vi "ClientIndividualUDP.vi"(0 "UDP Connection ID":refnum<k16>, 1 "Rover Inputs":cluster{"Left PWM":i32, "Right PWM":i32}={"Left PWM"=1500, "Right PWM"=1500}, 2 "Remote Port #":i32=61540, 3 "error in (no error)":errorcluster, 4 "Robot Symbol":string) -> (5 "connection ID out":refnum<k16>, 6 "Robot Heading":i32, 7 "error out":errorcluster)   [LabVIEW 2012]
panel:
  out "concatenated string":string
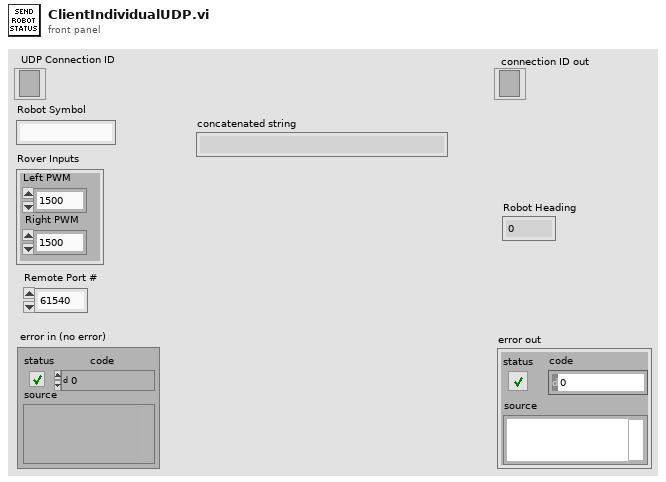
[diagram p1: front panel]
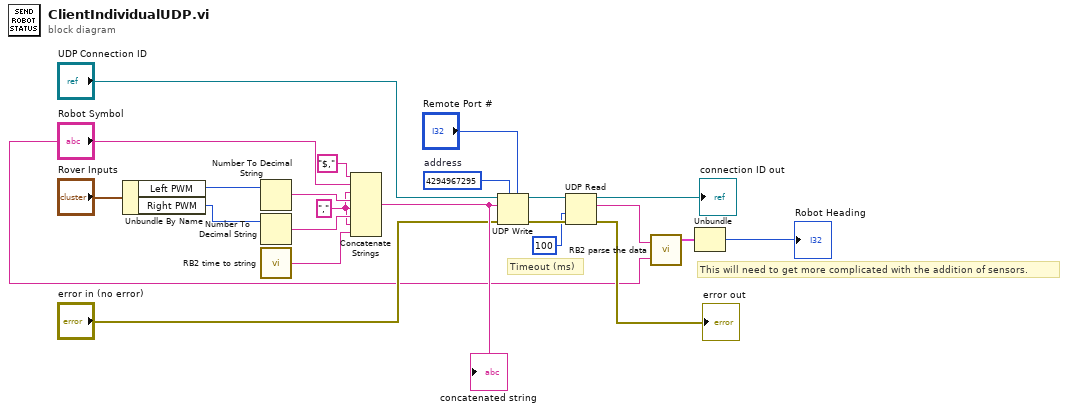
[diagram p0: block diagram]
diagram:
  w15 = u32 4294967295  # address
  w1 = "," ("string")
  # "Timeout (ms)"
  # "This will need to get more complicated with the addition of sensors."
  n1 = Unbundle By Name("Rover Inputs") -> ("Left PWM"=w21:i32, "Right PWM"=w20:i32)
  n2 = Number To Decimal String(number=w21) -> (decimal integer string=w18:string)  [unwired: 1 in]
  n3 = Number To Decimal String(number=w20) -> (decimal integer string=w19:string)  [unwired: 1 in]
  n4 = call "RB2 time to string.vi"() -> ("time string"=w17:string)  [unwired: 1 in]
  n5 = Concatenate Strings("$," ("string"), "Robot Symbol", w1, w18, w1, w19, w1, w17) -> (w16:string)
  "concatenated string" <- w16
  n6 = UDP Write(address=w15, port or service name="Remote Port #", connection ID="UDP Connection ID", data in=w16, 8:"error in (no error)") -> (error out=w10:errorcluster, 3:w11:refnum<k16>)  [unwired: 1 in]
  n7 = UDP Read(connection ID=w11, timeout ms (25000)=100, 8:w10) -> (data out=w7:string, error out=→"error out":errorcluster, 3:→"connection ID out":refnum<k16>)  [unwired: 1 in, 2 out]
  n8 = call "RB2 parse the data.vi"("Nav String"=w7, "Jeep"="Robot Symbol") -> ("Jeep Data"=w6:cluster{"Header":string, i32, i32})  [unwired: 2 out]
  n9 = Unbundle(w6) -> (→"Robot Heading":i32)  [unwired: 2 out]
